vi "Match_Cal STD.vi"(7 "Condition Default":string[][](array[string]), 9 "Data 2 in":string[][](array[string]), 10 "Data in":string[][][](array[string]), 11 "Cal STD":string[][][](array[string])) -> (1 "Data 2 Out":string[](array[string]), 2 "Data Out":string[][](array[string]), 3 "Cal STD":string[][](array[string]))   [LabVIEW 2020]
doc: "※ 명목값 index \"1\"\n 명목단위 index \"2\""
panel:
  # "※ Cal STD 명목값 index \"1\", 단위 index \"2\""
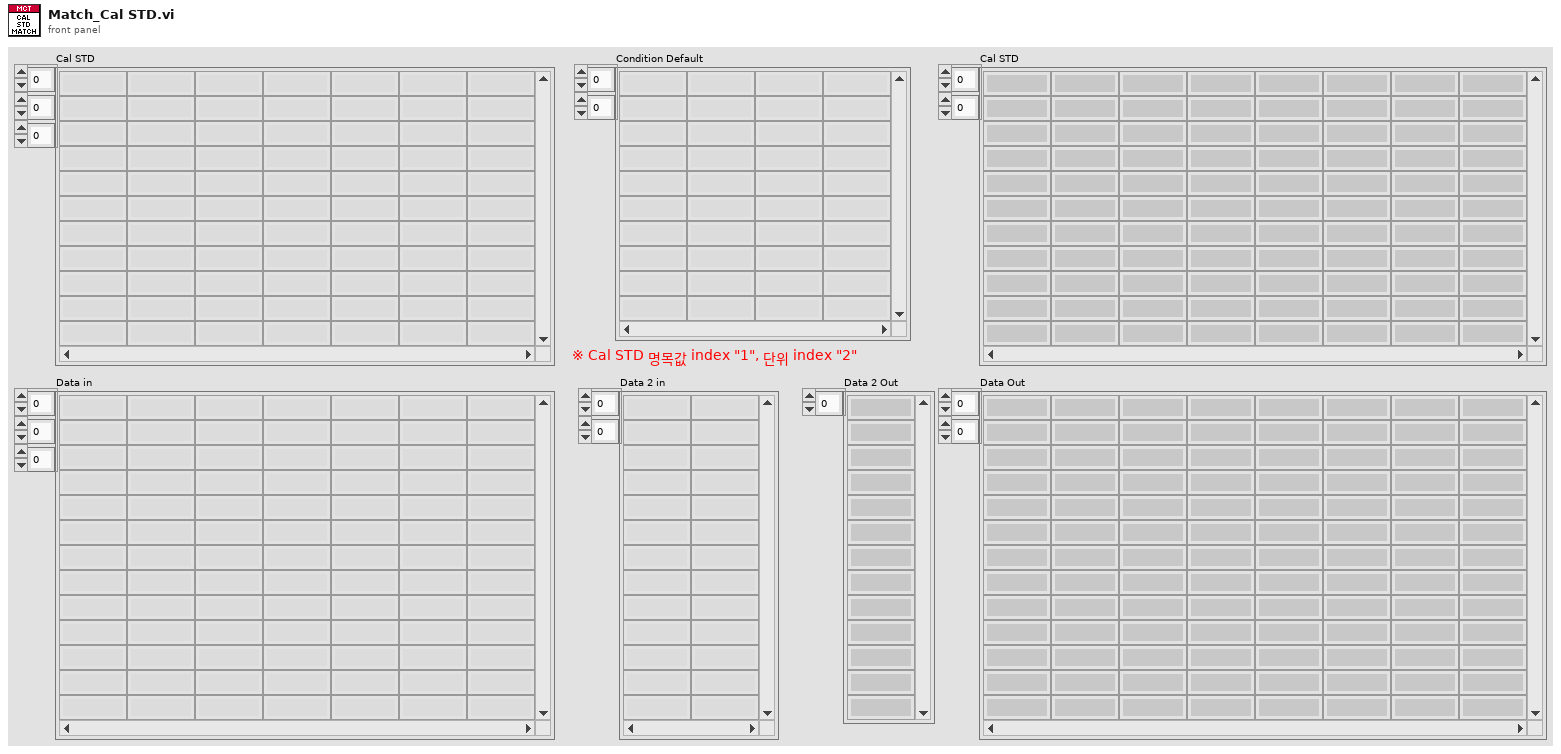
[diagram p1: front panel]
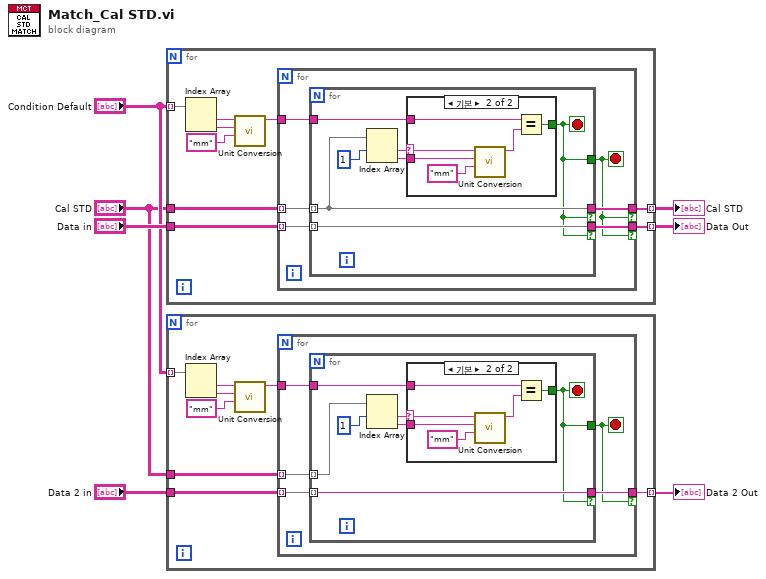
[diagram p0: block diagram]
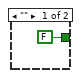
[diagram p2: hidden frame]
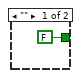
[diagram p3: hidden frame]
diagram:
  n1 = for {
    tunnel: "Condition Default" -> [w16] mode=indexing
    tunnel: "Cal STD" -> [w12]
    tunnel: [w10] -> w7 mode=indexing
    tunnel: "Data in" -> [w9]
    tunnel: [w8] -> w5 mode=indexing
    n2 = Index Array(array=w16) -> (element #1=w15:string, element #2=w14:string)  [unwired: 2 in]
    n3 = call "Unit Conversion.vi"("환산단위"="mm", "입력단위"=w14, "입력값"=w15) -> ("환산값 (string)"=w11:string)  [unwired: 3 in, 5 out]
    n4 = for {
      tunnel: w12 -> [w21] mode=indexing
      tunnel: w11 -> [w22]
      tunnel: [w20] -> w10 if=w17
      tunnel: w9 -> [w19] mode=indexing
      tunnel: [w18] -> w8 if=w17
      stop <- w17 stop-if-true
      n5 = for {
        tunnel: w21 -> [w27] mode=indexing
        tunnel: w22 -> [w28]
        tunnel: [w27] -> w20 if=w23
        tunnel: [w23] -> w17
        tunnel: w19 -> [w26] mode=indexing
        tunnel: [w26] -> w18 if=w23
        stop <- w23 stop-if-true
        n6 = Index Array(array=w27, index #1=1 ("명목값 인덱스")) -> (element #1=w24:string, element #2=w29:string)  [unwired: 1 in]
        n7 = case shown="기본" w24 {
          selector: w24 -> [_ w31]
          tunnel: w29 -> [_ w35]
          tunnel: w28 -> [_ w34]
          tunnel: [FALSE w32] -> w23
          frame "" {
          }
          frame Default {
            n8 = call "Unit Conversion.vi"("환산단위"="mm", "입력단위"=w35, "입력값"=w31) -> ("환산값 (string)"=w33:string)  [unwired: 3 in, 5 out]
            n9 = Equal?(x=w34, y=w33) -> (x = y?=w32:bool)
          }
        }
      }
    }
  }
  "Data Out" <- w5
  "Cal STD" <- w7
  n10 = for {
    tunnel: "Condition Default" -> [w44] mode=indexing
    tunnel: "Cal STD" -> [w40]
    tunnel: "Data 2 in" -> [w38]
    tunnel: [w37] -> w1 mode=indexing
    n11 = Index Array(array=w44) -> (element #1=w43:string, element #2=w42:string)  [unwired: 2 in]
    n12 = call "Unit Conversion.vi"("환산단위"="mm", "입력단위"=w42, "입력값"=w43) -> ("환산값 (string)"=w39:string)  [unwired: 3 in, 5 out]
    n13 = for {
      tunnel: w40 -> [w48] mode=indexing
      tunnel: w39 -> [w49]
      tunnel: w38 -> [w47] mode=indexing
      tunnel: [w46] -> w37 if=w45
      stop <- w45 stop-if-true
      n14 = for {
        tunnel: w48 -> [w54] mode=indexing
        tunnel: w49 -> [w55]
        tunnel: [w50] -> w45
        tunnel: w47 -> [w53] mode=indexing
        tunnel: [w53] -> w46 if=w50
        stop <- w50 stop-if-true
        n15 = Index Array(array=w54, index #1=1 ("명목값 인덱스")) -> (element #1=w51:string, element #2=w56:string)  [unwired: 1 in]
        n16 = case shown="기본" w51 {
          selector: w51 -> [_ w58]
          tunnel: w56 -> [_ w62]
          tunnel: w55 -> [_ w61]
          tunnel: [FALSE w59] -> w50
          frame "" {
          }
          frame Default {
            n17 = call "Unit Conversion.vi"("환산단위"="mm", "입력단위"=w62, "입력값"=w58) -> ("환산값 (string)"=w60:string)  [unwired: 3 in, 5 out]
            n18 = Equal?(x=w61, y=w60) -> (x = y?=w59:bool)
          }
        }
      }
    }
  }
  "Data 2 Out" <- w1
